vi "Enable_Disable Conrols.vi"(10 "Controls to Disable":refnum<vi>[](array[refnum]), 11 "Controls to Enable":refnum<vi>[](array[refnum])) -> ()   [LabVIEW 2019]
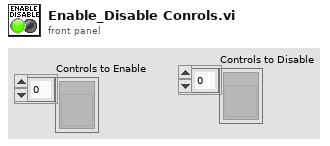
[diagram p1: front panel]
types:
  T1 = enum8{"Enabled", "Disabled", "Disabled and Grayed Out"}
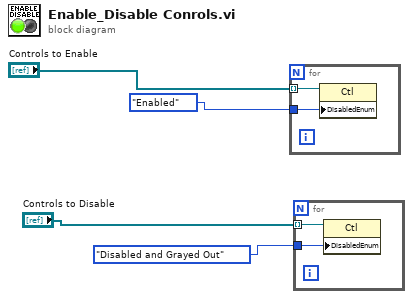
[diagram p0: block diagram]
diagram:
  n1 = for {
    tunnel: "Controls to Enable" -> [w6] mode=indexing
    tunnel: T1."Enabled" ("t") -> [w5]
    n2 = property class="Ctl"(reference=w6, "DisabledEnum"=w5) -> ()  [unwired: 1 in, 2 out]
  }
  n3 = for {
    tunnel: "Controls to Disable" -> [w8] mode=indexing
    tunnel: T1."Disabled and Grayed Out" ("Disabled") -> [w7]
    n4 = property class="Ctl"(reference=w8, "DisabledEnum"=w7) -> ()  [unwired: 1 in, 2 out]
  }
